vi "Const_Dapper.vi"() -> (0 "SQLMapper":refnum<class "SqlMapper.lvclass">)   [LabVIEW 2020]
uses:
  <vilib>/Viviota/shared/ORM_Dapper.lvlibp
  <vilib>/Viviota/shared/ORM.lvlibp/ORM/SqlMapper/SqlMapper.lvclass
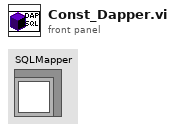
[diagram p1: front panel]
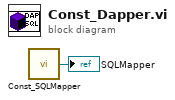
[diagram p0: block diagram]
diagram:
  n1 = call <vilib>:"Const_SQLMapper.vi"() -> ("SQLMapper"=→"SQLMapper":refnum<class "SqlMapper.lvclass">)
